vi "Scheduler.AddTask.vi"(4 "Data 2":variant, 5 "Recurring":bool, 6 "Data1":variant, 7 "Interval(s)":dbl=1.0 format="%#_13g", 8 "Error In":errorcluster, 9 "Task Name":string, 10 "Sched Name":string, 11 "Q In":refnum<queue>) -> (0 "Error Out":errorcluster, 3 "Q Out":refnum<queue>)   [LabVIEW 2024, in "EQMF.lvlib" / "Scheduler.lvlib"]
uses:
  Scheduler.lvlib
  Queues/Q.Element.ctl
  _Private/Scheduler.Item.ctl
  Queues/Queue Utils.lvlib
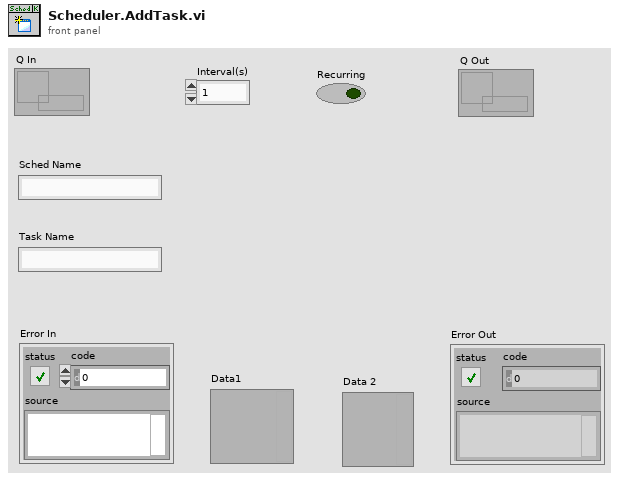
[diagram p1: front panel]
types:
  T1 = typedef "EQMF.lvlib/Scheduler.lvlib/Scheduler.Item.ctl" = cluster{"Name":string, "Start Time(s)":dbl, "Interval(s)":dbl, "Recurring":bool, "Q In":refnum<queue>, "Q.Element":T2}
  T2 = typedef "EQMF.lvlib/Queue Utils.lvlib/Q.Element.ctl" = cluster{"Cmd":string, "Sub":string, "Data1":variant, "Data2":variant}
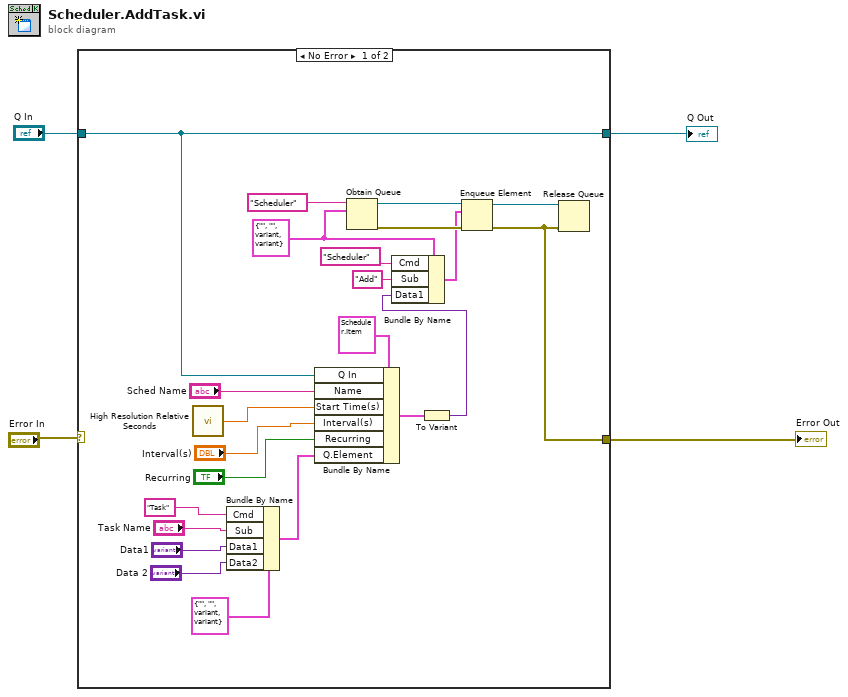
[diagram p0: block diagram]
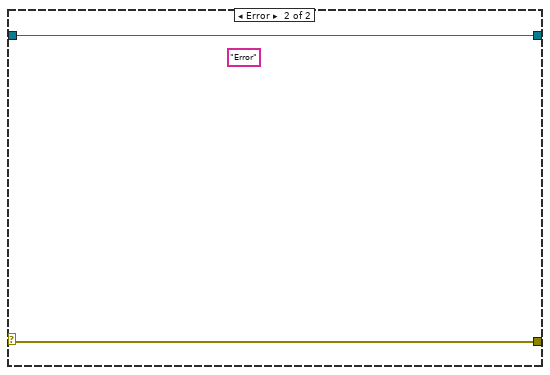
[diagram p2: hidden frame]
diagram:
  n1 = case shown="No Error" "Error In" {
    selector: "Error In" -> [_ w29]
    tunnel: "Q In" -> [w5 w28]
    tunnel: [w24 w29] -> w2
    tunnel: [w5 w28] -> w1
    frame No Error {
      w14 = T2 {"Cmd"="", "Sub"="", "Data1"=variant, "Data2"=variant} ("element")
      n2 = call <vilib>:"High Resolution Relative Seconds.vi"() -> ("relative seconds"=w9:dbl)
      n3 = Bundle By Name(cluster=T2 {"Cmd"="", "Sub"="", "Data1"=variant, "Data2"=variant} ("element"), "Cmd"="Task", "Sub"="Task Name", "Data1"="Data1", "Data2"="Data 2") -> (w18:T2)
      n4 = Bundle By Name(cluster=T1 {"Name"="", "Start Time(s)"=0.0, "Interval(s)"=0.0, "Recurring"=FALSE, "Q In"=refnum, "Q.Element"={"Cmd"="", "Sub"="", "Data1"=variant, "Data2"=variant}}, "Q In"=w5, "Name"="Sched Name", "Start Time(s)"=w9, "Interval(s)"="Interval(s)", "Recurring"="Recurring", "Q.Element"=w18) -> (w8:T1)
      n5 = Obtain Queue(name (unnamed)="Scheduler" ("Cmd"), element data type=w14) -> (queue out=w26:refnum<queue>, error out=w25:errorcluster)  [unwired: 3 in, 1 out]
      n6 = To Variant(anything=w8) -> (Variant=w7:variant)
      n7 = Bundle By Name(cluster=w14, "Cmd"="Scheduler", "Sub"="Add" ("Cmd"), "Data1"=w7) -> (w12:T2)
      n8 = Enqueue Element(queue=w26, element=w12, error in (no error)=w25) -> (queue out=w23:refnum<queue>, error out=w24:errorcluster)  [unwired: 1 in, 1 out]
      n9 = Release Queue(queue=w23, error in (no error)=w24) -> ()  [unwired: 1 in, 3 out]
    }
    frame Error {
      (unwired) "Error"
    }
  }
  "Q Out" <- w1
  "Error Out" <- w2
